vi "TSLIN_SetNodeFuntionType.vi"(9 "set_node_funtiontype":i32(ring) items=["MasterNode", "SlaveNode", "MonitorNote"], 10 "AAppChannel":i32(ring) items=["CHN1", "CHN2", "CHN3", "CHN4", "CHN5", "CHN6", "CHN7", "CHN8", "CHN9", "CHN10", "CHN11", "CHN12", "CHN13", "CHN14", "CHN15", "CHN16", "CHN17", "CHN18", "CHN19", "CHN20", "CHN21", "CHN22", "CHN23", "CHN24", "CHN25", "CHN26", "CHN27", "CHN28", "CHN29", "CHN30", "CHN31", "CHN32"], 11 "路径输入":path) -> (3 "路径输出":path)   [LabVIEW 2019]
panel:
  out "tslin_set_node_funtiontype":i32
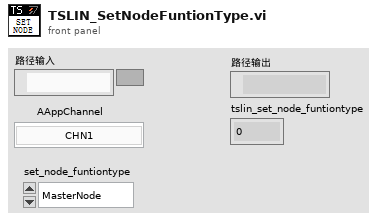
[diagram p1: front panel]
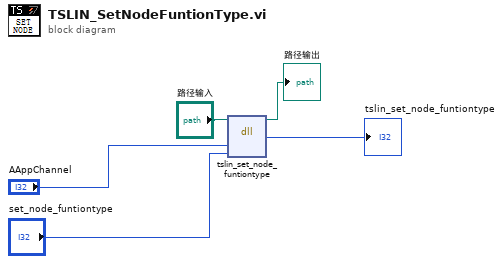
[diagram p0: block diagram]
diagram:
  n1 = dll-call lib="PTH2@abs EDemo同星TSCAN_V1.4_20220301ConfigTSMaster.dll" fn="tslin_set_node_funtiontype"(path in="路径输入", "AChnIdx"="AAppChannel", "AFunctionType"="set_node_funtiontype") -> (path out=→"路径输出":path, "tslin_set_node_funtiontype"=→"tslin_set_node_funtiontype":i32)  [unwired: 4 in, 1 out]
